vi "02escribe_lee_placa.vi"(0 "cantmedic":u8, 1 "comando":string, 2 "IP":string, 3 "Puerto":u16, 4 "Time Out":u16) -> (5 "DATA":string, 6 "error out":errorcluster)   [LabVIEW 2010]
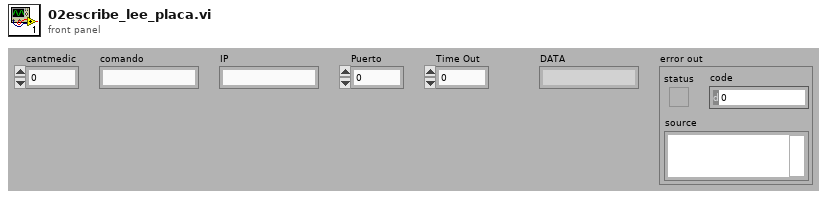
[diagram p1: front panel]
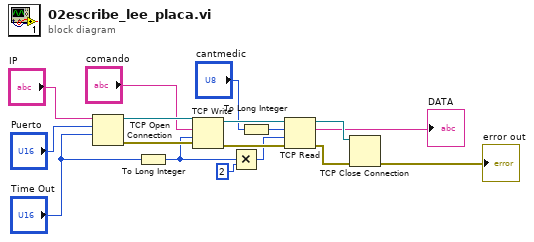
[diagram p0: block diagram]
diagram:
  n1 = TCP Open Connection(address="IP", remote port or service name="Puerto", timeout ms (60000)="Time Out") -> (connection ID=w10:refnum<k5>, error out=w11:errorcluster)  [unwired: 2 in]
  n2 = To Long Integer(number="Time Out") -> (32bit integer=w8:i32)
  n3 = TCP Write(connection ID=w10, data in="comando", error in (no error)=w11, 9:w8) -> (connection ID out=w3:refnum<k5>, error out=w7:errorcluster)  [unwired: 1 out]
  n4 = Multiply(x=w8, y=2) -> (x*y=w5:i32)
  n5 = To Long Integer(number="cantmedic") -> (32bit integer=w9:i32)
  n6 = TCP Read(connection ID=w3, bytes to read=w9, error in (no error)=w7, 9:w5) -> (connection ID out=w12:refnum<k5>, data out=→"DATA":string, error out=w13:errorcluster)  [unwired: 1 out]
  n7 = TCP Close Connection(connection ID=w12, error in (no error)=w13) -> (error out=→"error out":errorcluster)  [unwired: 1 in, 1 out]
